vi "Tell.vi"(10 "Msg":refnum<class "Msg.lvclass">, 11 "Queue Transport in":refnum<class "Queue Transport.lvclass">) -> (0 "Error out":errorcluster)   [LabVIEW 2025, in "jettl.lvlib" / "Transport.lvlib" / "Queue.lvlib" / "Queue Transport.lvclass"]
uses:
  Queue Transport.lvclass
  Msg/Msg.lvclass
  Queue Transport.lvclass/Queue Transport.ctl
  Teller/Teller.lvclass
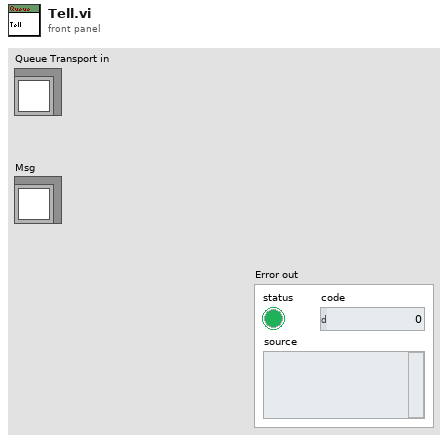
[diagram p1: front panel]
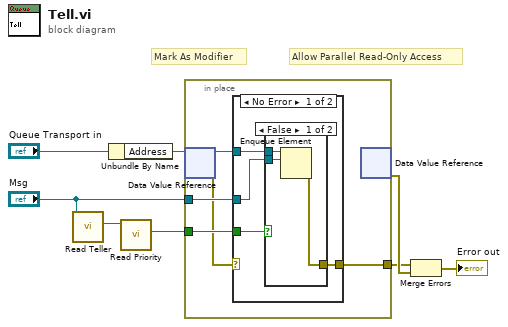
[diagram p0: block diagram]
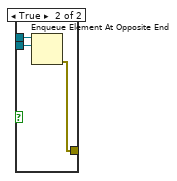
[diagram p2: hidden frame]
diagram:
  # "Allow Parallel Read-Only Access"
  # "Mark As Modifier"
  n1 = call-dynamic "Read Teller.vi"("Msg in"="Msg") -> ("Teller"=w3:refnum<class "Teller.lvclass">)  [unwired: 10 in]
  n2 = Unbundle By Name("Queue Transport in") -> ("Address"=w7:refnum<data-value>)
  n3 = call-dynamic "Read Priority.vi"("Teller in"=w3) -> ("Priority"=w1:bool)  [unwired: 10 in]
  n4 = in-place {
    in-place-border: [w13] -> w4
    in-place-border: "Msg" -> [w12]
    in-place-border: w1 -> [w11]
    n5 = in-place-dvr #1(w7) -> (w10:refnum<queue>, w9:errorcluster)
    n6 = case shown="No Error" w9 {
      selector: w9 -> [_ w24]
      tunnel: [w17 w24] -> w13
      tunnel: w12 -> [w16 _]
      tunnel: w11 -> [w15 _]
      tunnel: w10 -> [w14 _]
      frame No Error {
        n7 = case shown="False" w15 {
          tunnel: w14 -> [w20 w23]
          tunnel: [w19 w21] -> w17
          tunnel: w16 -> [w18 w22]
          frame False {
            n8 = Enqueue Element(queue=w20, element=w18) -> (error out=w19:errorcluster)  [unwired: 2 in, 2 out]
          }
          frame True {
            n9 = Enqueue Element At Opposite End(queue=w23, element=w22) -> (error out=w21:errorcluster)  [unwired: 2 in, 2 out]
          }
        }
      }
      frame Error {
      }
    }
    n10 = in-place-dvr #1() -> (w5:errorcluster)  [unwired: 1 in, 1 out]
  }
  n11 = Merge Errors(w4, w5) -> (→"Error out":errorcluster)
